vi "Day 1 - Calorie Counting.vi"() -> ()   [LabVIEW 2020, in "AoC 2022.lvlib"]
uses:
  AoC 2022.lvlib
panel:
  out "Puzzle Part-2 Answer":string
  out "Puzzle Answer":string
  in  "Puzzle Input":string
  # "Enter the Puzzle Input and run the VI"
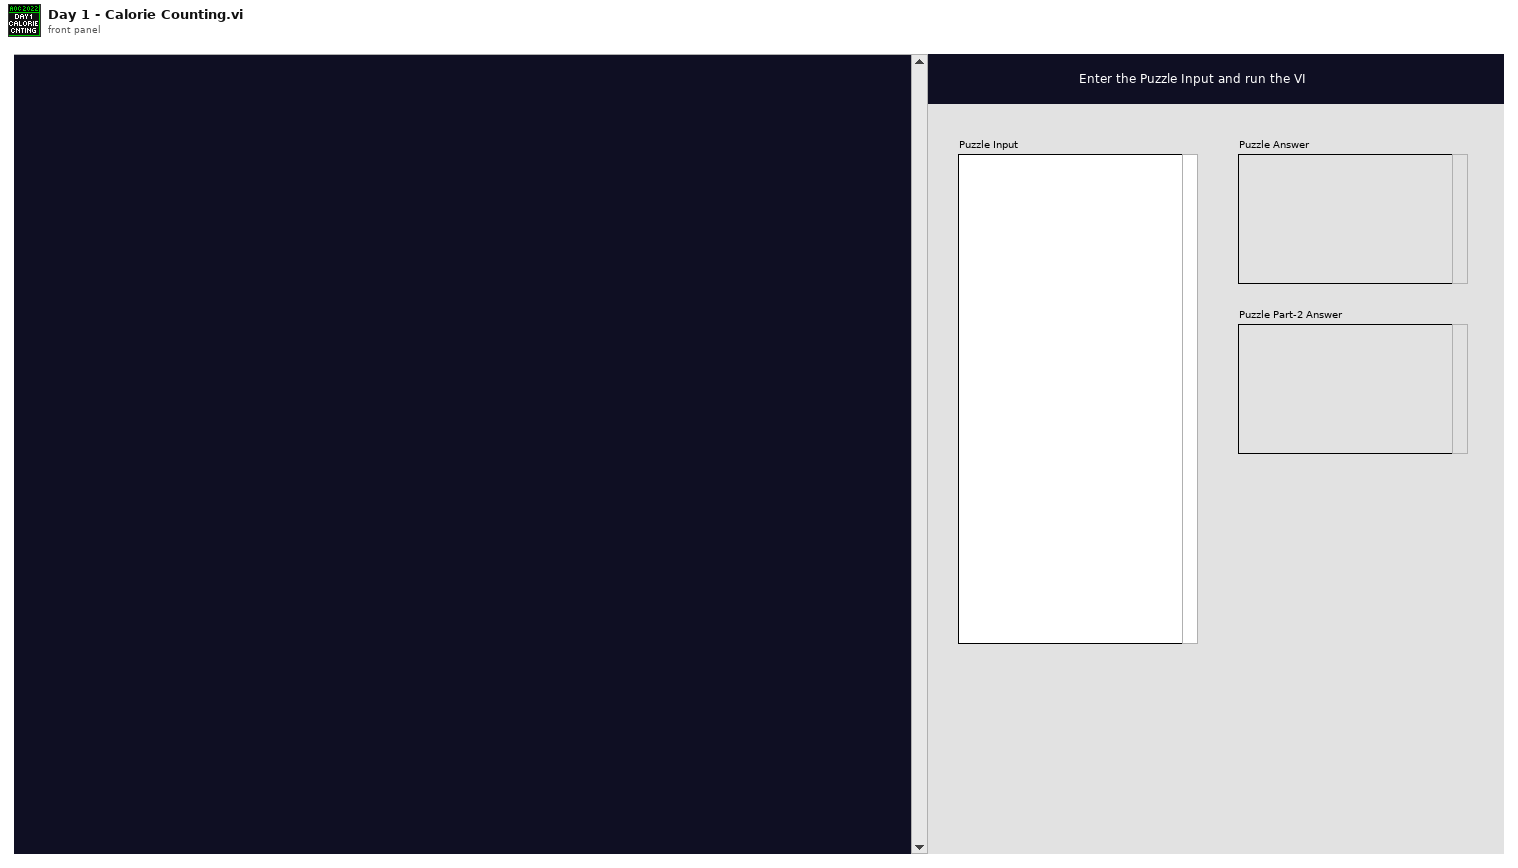
[diagram p1: front panel]
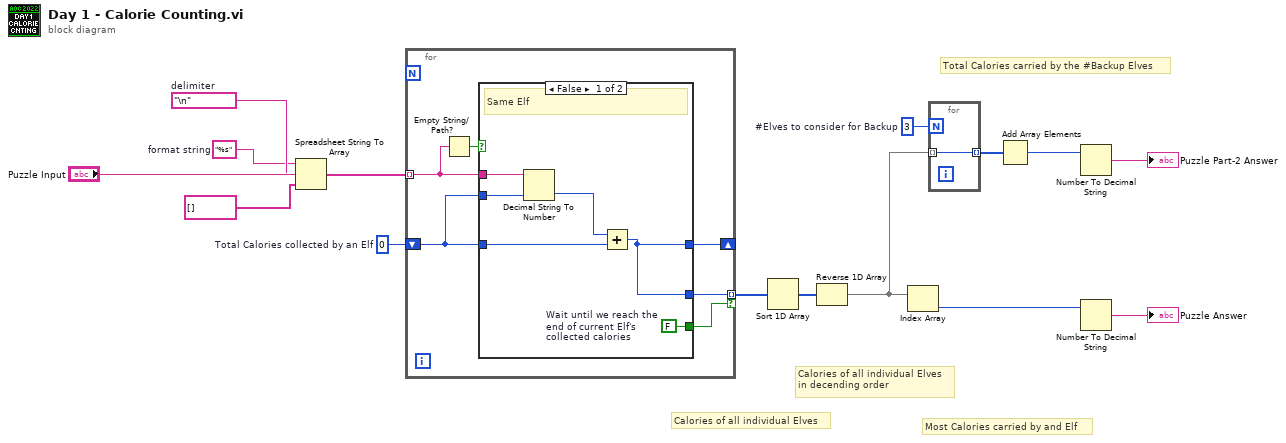
[diagram p0: block diagram]
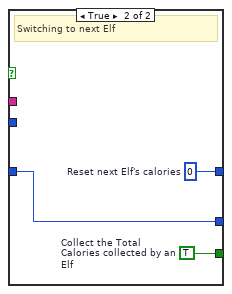
[diagram p2: hidden frame]
diagram:
  w4 = 3  # #Elves to consider for Backup
  w10 = u32 0  # Total Calories collected by an Elf
  w13 = "%s"  # format string
  w14 = "\n"  # delimiter
  # "Total Calories carried by the #Backup Elves"
  # "Most Calories carried by and Elf"
  # "Calories of all individual Elves\nin decending order"
  # "Calories of all individual Elves"
  n1 = Spreadsheet String To Array(delimiter (Tab)=w14, format string=w13, spreadsheet string="Puzzle Input", array type (2D Dbl)=string[] []) -> (array=w11:string[])
  n2 = for {
    tunnel: w11 -> [w21] mode=indexing
    shift-right: [w18] -> _
    shift-left: w10 -> [w19]
    tunnel: [w17] -> w7 mode=indexing if=w16
    n3 = Empty String/Path?(string/path=w21) -> (empty?=w20:bool)
    n4 = case shown="False" w20 {
      tunnel: w19 -> [w27 _]
      tunnel: w21 -> [w26 _]
      tunnel: w19 -> [w24 w29]
      tunnel: [w22 w30] -> w18
      tunnel: [w22 w29] -> w17
      tunnel: [w23 w28] -> w16
      frame False {
        w23 = FALSE  # Wait until we reach the end of current Elf's collected calories
        # "Same Elf"
        n5 = Decimal String To Number(string=w26, default (0L)=w27) -> (number=w25:u32)  [unwired: 1 in, 1 out]
        n6 = Add(x=w25, y=w24) -> (x+y=w22:u32)
      }
      frame True {
        w28 = TRUE  # Collect the Total Calories collected by an Elf
        w30 = u32 0  # Reset next Elf's calories
        # "Switching to next Elf"
      }
    }
  }
  n7 = Sort 1D Array(array=w7) -> (sorted array=w6:u32[])
  n8 = Reverse 1D Array(array=w6) -> (reversed array=w5:u32[])
  n9 = Index Array(array=w5) -> (element=w8:u32)  [unwired: 1 in]
  n10 = for {
    N: w4 -> [_]
    tunnel: w5 -> [w31] mode=indexing
    tunnel: [w31] -> w3 mode=indexing
  }
  n11 = Add Array Elements(numeric array=w3) -> (sum=w2:u32)
  n12 = Number To Decimal String(number=w2) -> (decimal integer string=→"Puzzle Part-2 Answer":string)  [unwired: 1 in]
  n13 = Number To Decimal String(number=w8) -> (decimal integer string=→"Puzzle Answer":string)  [unwired: 1 in]
